vi "Find Value from Key (JSON).vi"(8 "error in (no error)":errorcluster, 10 "key":string, 11 "JSON Object in":refnum<class "JSON Object.lvclass">) -> (0 "error out":errorcluster, 2 "value":refnum<class "JSON Datatype.lvclass">, 3 "JSON Object out":refnum<class "JSON Object.lvclass">)   [LabVIEW 2017, in "LVJSON.lvlib" / "JSON Object.lvclass"]
uses:
  JSON Object.lvclass
  JSON Datatype/JSON Datatype.lvclass
  JSON Object.lvclass/JSON Object.ctl
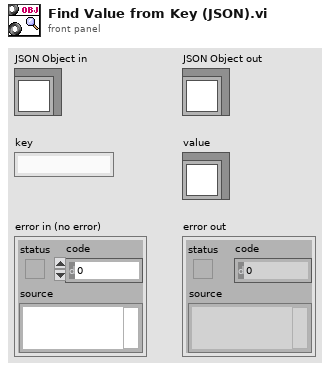
[diagram p1: front panel]
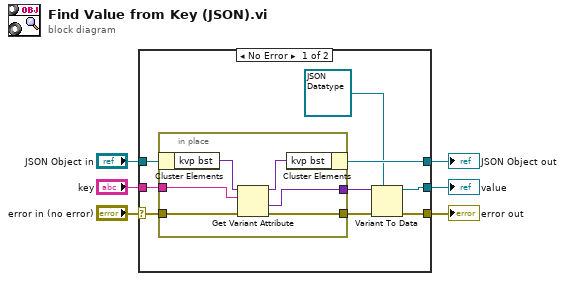
[diagram p0: block diagram]
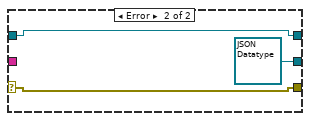
[diagram p2: hidden frame]
diagram:
  n1 = case shown="No Error" "error in (no error)" {
    selector: "error in (no error)" -> [w11 w24]
    tunnel: [w9 w24] -> w5
    tunnel: [w13 w23] -> w3
    tunnel: "JSON Object in" -> [w15 w23]
    tunnel: "key" -> [w14 _]
    tunnel: [w7 refnum<class "JSON Datatype.lvclass"> refnum ("value")] -> w1
    frame No Error {
      n2 = in-place {
        in-place-border: w14 -> [w19]
        in-place-border: [w18] -> w12
        in-place-border: w11 -> [w17]
        in-place-border: [w16] -> w10
        n3 = in-place-cluster #1(w15) -> ("kvp bst"=w21:variant)
        n4 = Get Variant Attribute(Variant=w21, name=w19, error in=w17) -> (duplicate Variant=w20:variant, value=w18:variant, error out=w16:errorcluster)  [unwired: 1 in, 1 out]
        n5 = in-place-cluster #1("kvp bst"=w20) -> (w13:refnum<class "JSON Object.lvclass">)
      }
      n6 = Variant To Data(error in=w10, type=refnum<class "JSON Datatype.lvclass"> refnum ("JSON Datatype.lvclass"), Variant=w12) -> (data=w7:refnum<class "JSON Datatype.lvclass">, error out=w9:errorcluster)
    }
    frame Error {
    }
  }
  "error out" <- w5
  "JSON Object out" <- w3
  "value" <- w1
